vi "Resample_By_N.vi"(1 "Resample Factor":i32=1 min=1, 2 "Array In":dbl[](array[numeric])) -> (0 "Array Out":dbl[](array[numeric]))   [LabVIEW 2011]
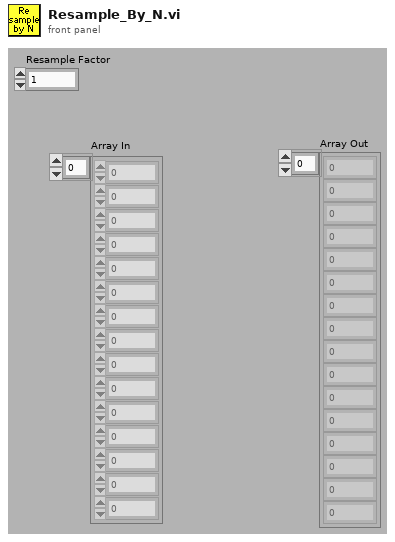
[diagram p1: front panel]
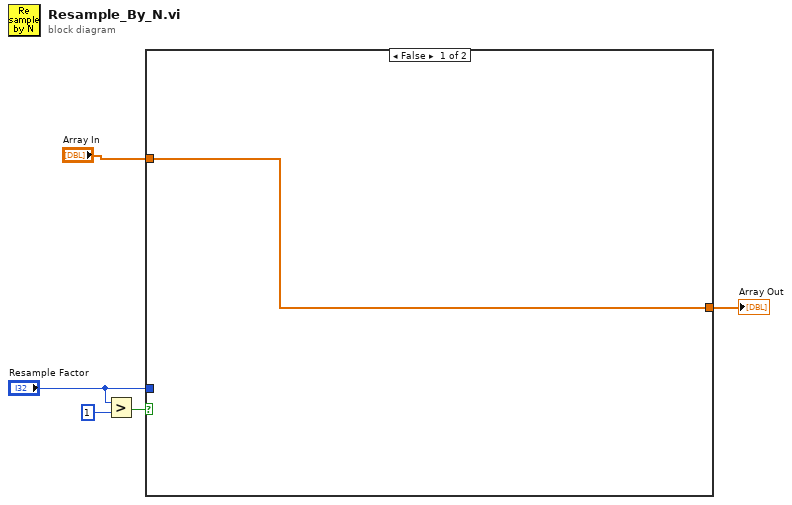
[diagram p0: block diagram]
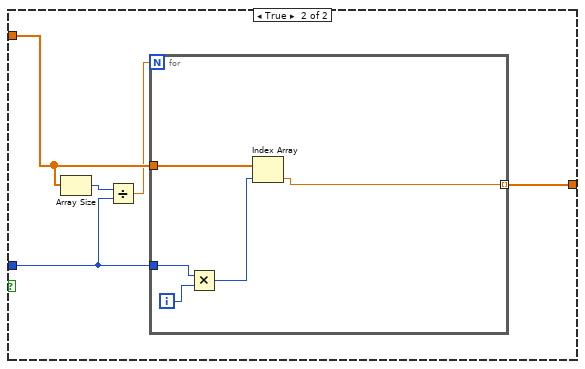
[diagram p2: hidden frame]
diagram:
  n1 = Greater?(x="Resample Factor", y=1) -> (0:w4:bool)
  n2 = case shown="False" w4 {
    tunnel: "Resample Factor" -> [_ w9]
    tunnel: "Array In" -> [w6 w11]
    tunnel: [w6 w7] -> w1
    frame False {
    }
    frame True {
      n3 = Array Size(array=w11) -> (size(s)=w10:i32)
      n4 = Divide(x=w10, y=w9) -> (x/y=w8:dbl)
      n5 = for {
        N: w8 -> [_]
        tunnel: w9 -> [w15]
        tunnel: w11 -> [w13]
        tunnel: [w12] -> w7 mode=indexing
        i -> [w16]
        n6 = Multiply(x=w15, y=w16) -> (x*y=w14:i32)
        n7 = Index Array(array=w13, index=w14) -> (element=w12:dbl)
      }
    }
  }
  "Array Out" <- w1
